vi "MTMount_getEvent_mountInPosition.vi"(8 "error in (no error)":errorcluster, 11 "logevent_mountInPosition_Ctl":T1) -> (0 "error out":errorcluster, 2 "function return":i32, 3 "logevent_mountInPosition_Ctl out":T1)   [LabVIEW 2018, in "SALLV_MTMount.lvlib"]
doc: "int MTMount_shm_getEvent_mountInPositionLV(MTMount_logevent_mountInPositionLV *logevent_mountInPosition_Ctl );"
uses:
  SALLV_MTMount.lvlib
  DataTypes/logevent_mountInPosition.ctl
  SALLV_MTMount.so
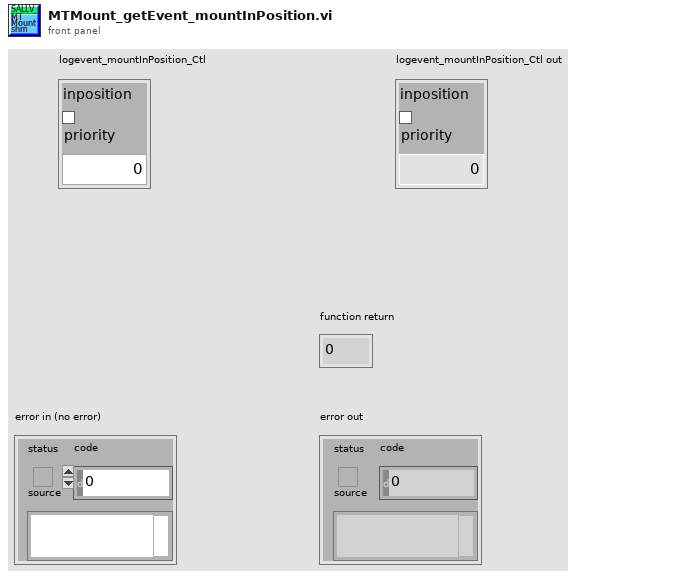
[diagram p1: front panel]
types:
  T1 = typedef "SALLV_MTMount.lvlib/logevent_mountInPosition.ctl" = cluster{"inposition":bool, "priority":i32}
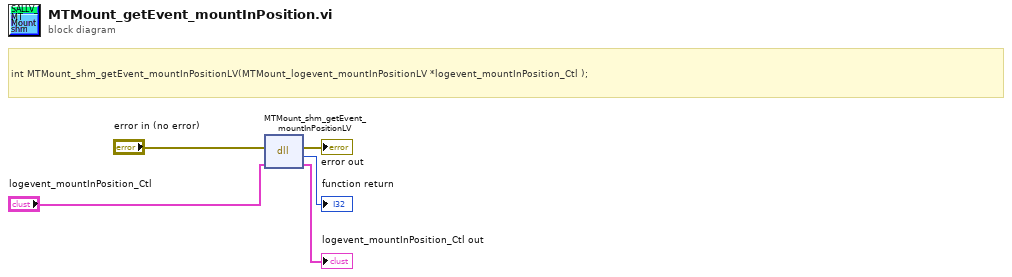
[diagram p0: block diagram]
diagram:
  # "int MTMount_shm_getEvent_mountInPositionLV(MTMount_logevent_mountInPositionLV *logevent_mountInPosition_Ctl );"
  n1 = dll-call lib="home/ttsai/Document/salApiMTMount/SALLV_MTMount/SALLV_MTMount.*" fn="MTMount_shm_getEvent_mountInPositionLV"(error in="error in (no error)", "logevent_mountInPosition_Ctl"="logevent_mountInPosition_Ctl") -> (error out=→"error out":errorcluster, →"function return":i32, "logevent_mountInPosition_Ctl"=→"logevent_mountInPosition_Ctl out":T1)  [unwired: 2 in, 1 out]
